vi "Manuele override - test.vi"() -> ()   [LabVIEW 2019]
panel:
  out "Meter":dbl(knob) scale=0.0..10.0
  in  "kruispunt":string
  out "bericht":string
  in  "STOP":bool
  in  "START":bool
  in  "stop 2":bool
  out "address":u32
  out "port":u16
  in  "stop":bool
  in  "vooruit":bool
  in  "achteruit":bool
  in  "links":bool
  in  "rechts":bool
  in  "linksvooruit":bool
  in  "rechtsvooruit":bool
  in  "rechtsachter":bool
  in  "linksachter":bool
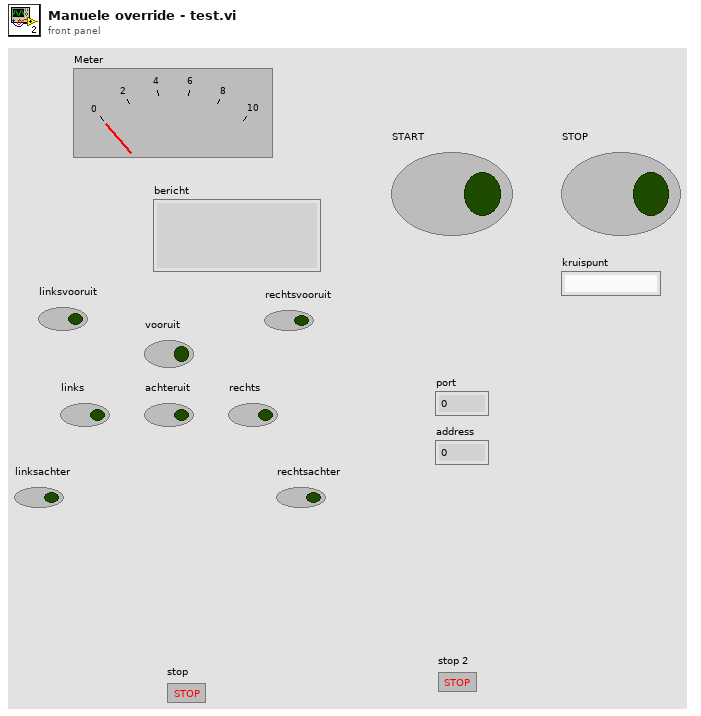
[diagram p1: front panel]
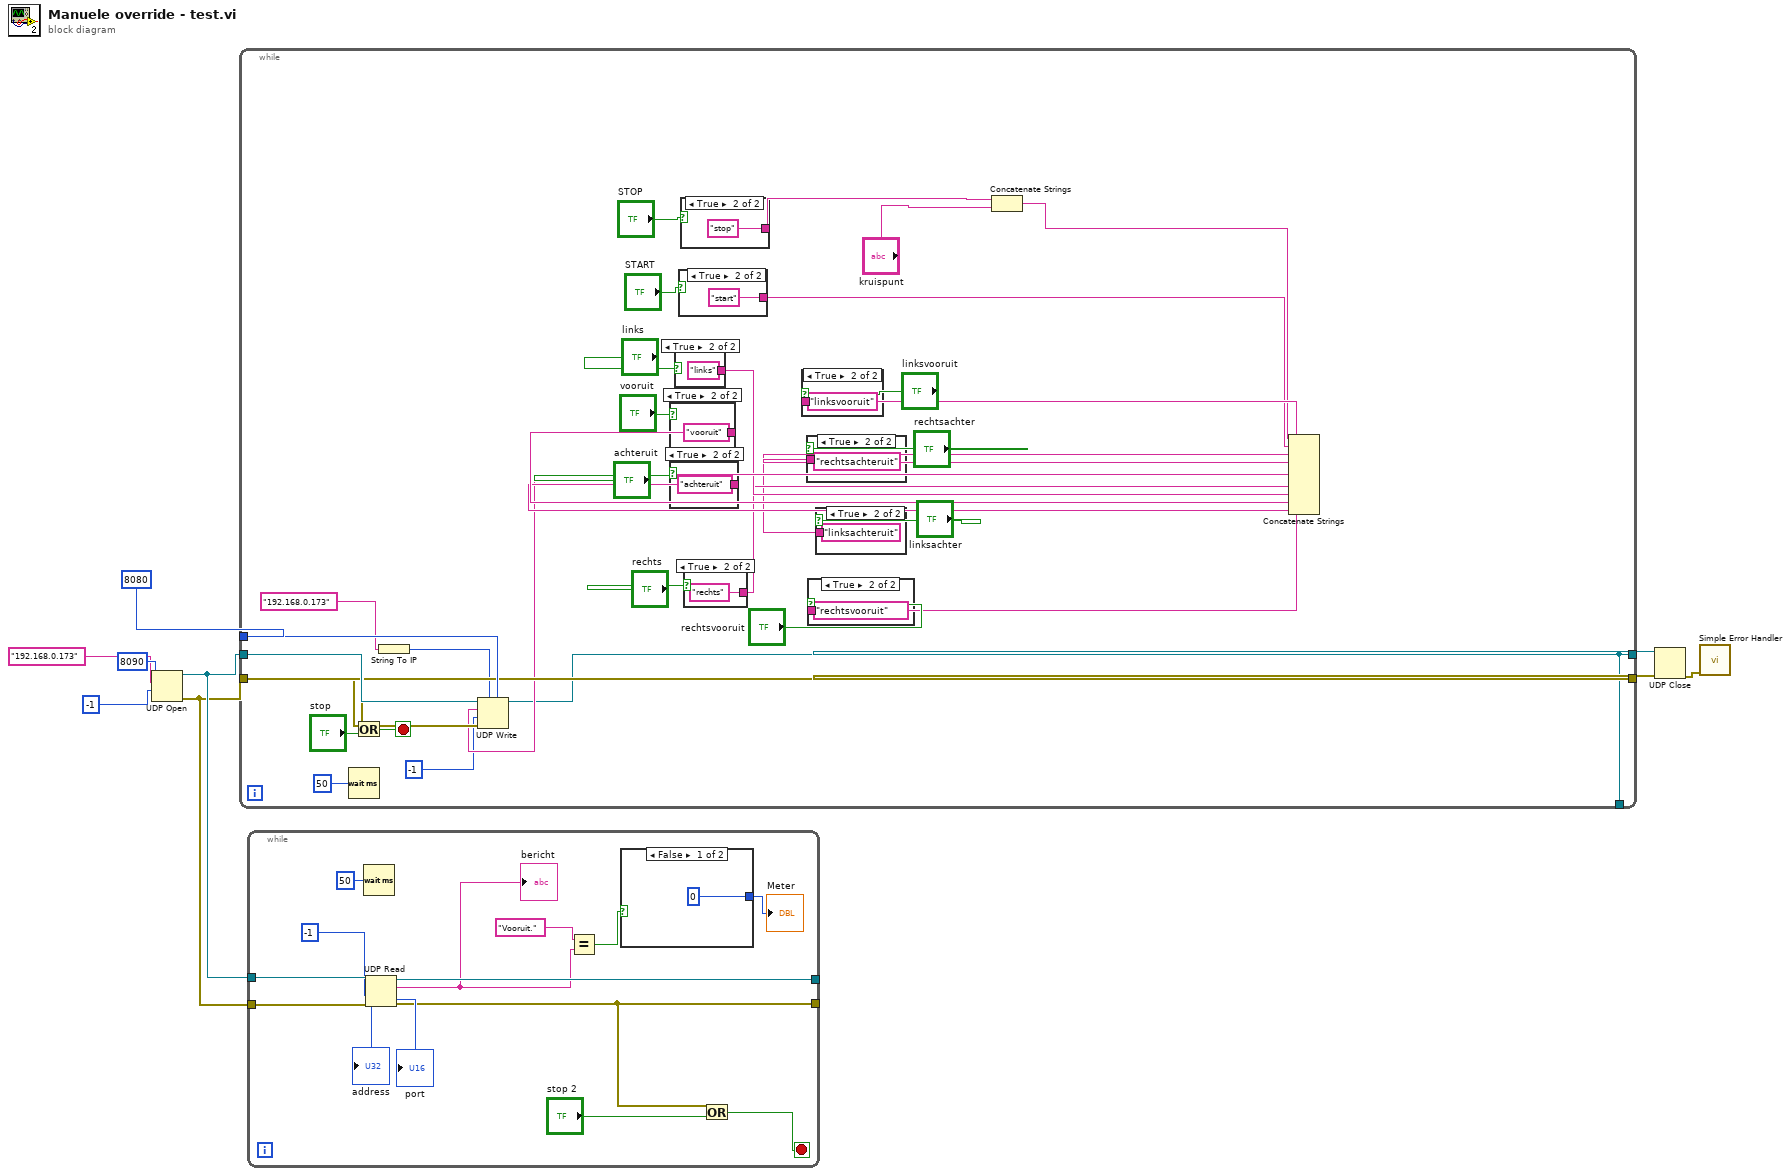
[diagram p0: block diagram]
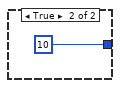
[diagram p2: hidden frame]
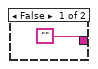
[diagram p3: hidden frame]
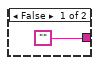
[diagram p4: hidden frame]
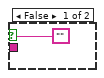
[diagram p5: hidden frame]
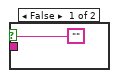
[diagram p6: hidden frame]
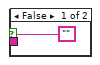
[diagram p7: hidden frame]
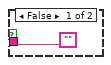
[diagram p8: hidden frame]
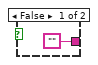
[diagram p9: hidden frame]
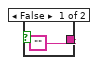
[diagram p10: hidden frame]
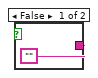
[diagram p11: hidden frame]
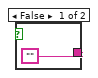
[diagram p12: hidden frame]
diagram:
  n1 = UDP Open(9:-1, 10:"192.168.0.173", 11:8090) -> (port=w5:refnum<k16>, 0:w4:errorcluster)  [unwired: 2 in, 1 out]
  n2 = while {
    tunnel: w5 -> [w43]
    tunnel: w4 -> [w42]
    tunnel: 8080 -> [w38]
    tunnel: [w19] -> w3
    tunnel: [w37] -> w7
    tunnel: [w19] -> _
    stop <- w40 stop-if-true
    n3 = Wait (ms)(milliseconds to wait=50) -> ()  [unwired: 1 out]
    n4 = String To IP(1:"192.168.0.173") -> (0:w30:u32)
    n5 = case shown="True" "vooruit" {
      tunnel: ["" "vooruit"] -> w34
      frame False {
      }
      frame True {
      }
    }
    n6 = case shown="True" "achteruit" {
      tunnel: ["" "achteruit"] -> w33
      frame False {
      }
      frame True {
      }
    }
    n7 = case shown="True" "links" {
      tunnel: ["" "links"] -> w29
      frame False {
      }
      frame True {
      }
    }
    n8 = case shown="True" "START" {
      tunnel: ["" "start"] -> w16
      frame False {
      }
      frame True {
      }
    }
    n9 = case shown="True" "STOP" {
      tunnel: ["" "stop"] -> w12
      frame False {
      }
      frame True {
      }
    }
    n10 = case shown="True" "rechts" {
      tunnel: ["" "rechts"] -> w27
      frame False {
      }
      frame True {
      }
    }
    n11 = case shown="True" "linksvooruit" {
      tunnel: ["" "linksvooruit"] -> w23
      frame False {
      }
      frame True {
      }
    }
    n12 = case shown="True" "rechtsachter" {
      tunnel: ["" "rechtsachteruit"] -> w21
      frame False {
      }
      frame True {
      }
    }
    n13 = case shown="True" "rechtsvooruit" {
      tunnel: ["" "rechtsvooruit"] -> w24
      frame False {
      }
      frame True {
      }
    }
    n14 = case shown="True" "linksachter" {
      tunnel: ["" "linksachteruit"] -> w20
      frame False {
      }
      frame True {
      }
    }
    n15 = Concatenate Strings(w12, "kruispunt") -> (w13:string)
    n16 = Concatenate Strings(w13, w16, w20, w21, w23, w24, w27, w29, w34, w33) -> (w32:string)
    n17 = UDP Write(address=w30, port or service name=w38, connection ID=w43, data in=w32, 8:w42, 9:-1) -> (error out=w37:errorcluster, 3:w19:refnum<k16>)
    n18 = Or(x=w37, y="stop") -> (x .or. y?=w40:bool)
  }
  n19 = while {
    tunnel: w5 -> [w77]
    tunnel: w4 -> [w76]
    tunnel: [w73] -> _
    tunnel: [w72] -> _
    stop <- w70 stop-if-true
    n20 = Wait (ms)(milliseconds to wait=u32 50) -> ()  [unwired: 1 out]
    n21 = UDP Read(connection ID=w77, timeout ms (25000)=-1, 8:w76) -> (data out=w68:string, error out=w72:errorcluster, 3:w73:refnum<k16>, 4:→"port":u16, 6:→"address":u32)  [unwired: 1 in]
    "bericht" <- w68
    n22 = Equal?(x="Vooruit.", y=w68) -> (x = y?=w66:bool)
    n23 = case shown="False" w66 {
      tunnel: [0 10] -> w65
      frame False {
      }
      frame True {
      }
    }
    "Meter" <- w65
    n24 = Or(x=w72, y="stop 2") -> (x .or. y?=w70:bool)
  }
  n25 = UDP Close(connection ID=w3, 8:w7) -> (error out=w6:errorcluster)  [unwired: 1 out]
  n26 = call <vilib>:"Simple Error Handler.vi"("error in (no error)"=w6) -> ()  [unwired: 4 in, 5 out]
